vi "Run Voicemeeter.vi"(8 "error in (no error)":errorcluster, 10 "Voicemeeter Type":T1=enum."Voicemeeter", 11 "VoiceMeeterRemote in":refnum<class "VoiceMeeterRemote.lvclass">) -> (0 "error out":errorcluster, 3 "VoiceMeeterRemote out":refnum<class "VoiceMeeterRemote.lvclass">)   [LabVIEW 2022 SP3, in "VoiceMeeterRemote.lvlib" / "VoiceMeeterRemote.lvclass"]
uses:
  VoiceMeeterRemote.lvclass
  Voicemeeter Type.ctl
  VoiceMeeterRemote.lvclass/VoiceMeeterRemote.ctl
  VoiceMeeterRemote.lvlib
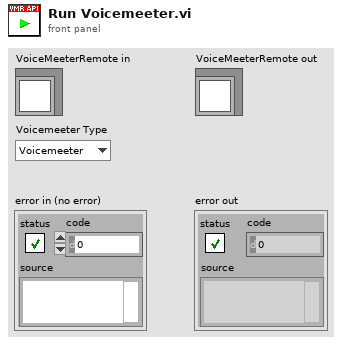
[diagram p1: front panel]
types:
  T1 = typedef "VoiceMeeterRemote.lvlib/Voicemeeter Type.ctl" = enum16{"Unknown", "Voicemeeter", "Banana", "Potato", "Potato x64"}
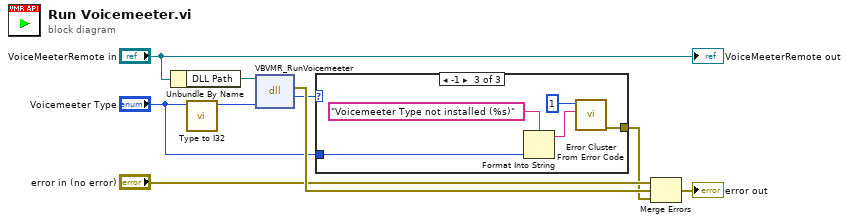
[diagram p0: block diagram]
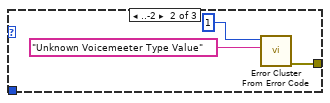
[diagram p3: hidden frame]
diagram:
  n1 = Unbundle By Name("VoiceMeeterRemote in") -> ("DLL Path"=w6:path)
  n2 = call "Type to I32.vi"("Voicemeeter Type"="Voicemeeter Type") -> ("Type I32"=w5:i32)  [unwired: 10 in]
  n3 = dll-call lib="C:/Program Files/National Instruments/LabVIEW 2022/user.lib/VoicemeeterRemote64/VoicemeeterRemote64.*" fn="VBVMR_RunVoicemeeter"(path in=w6, "vType"=w5) -> (error out=w9:errorcluster, "return type"=w4:i32)  [unwired: 3 in, 1 out]
  n4 = case shown="-1" w4 {
    tunnel: [_ w10 w16] -> w1
    tunnel: "Voicemeeter Type" -> [_ _ w14]
    frame 0, Default {
    }
    frame ..-2 {
      n5 = call <vilib>:"Error Cluster From Error Code.vi"("error message (\"\")"="Unknown Voicemeeter Type Value" ("error message (\"\")"), "error code (0)"=1) -> ("error out"=w10:errorcluster)  [unwired: 7 in]
    }
    frame -1 {
      n6 = Format Into String(format string="Voicemeeter Type not installed (%s)" ("error message (\"\")"), w14) -> (resulting string=w13:string)  [unwired: 2 in, 1 out]
      n7 = call <vilib>:"Error Cluster From Error Code.vi"("error message (\"\")"=w13, "error code (0)"=1) -> ("error out"=w16:errorcluster)  [unwired: 7 in]
    }
  }
  n8 = Merge Errors("error in (no error)", w9, w1) -> (→"error out":errorcluster)
  "VoiceMeeterRemote out" <- "VoiceMeeterRemote in"
